vi "GetDisplayName3.vi"(0 "XRef":T15, 1 "State In":T3={"Worker Library Path"=path "", "Block Label"="", "Types"=[], "Selections"=[], "Icon"={"image type"=0, "image depth"=0, "image"=[], "mask"=[], "colors"=[], "Rectangle"={"left"=0, "top"=0, "right"=0, "bottom"=0}}, "Errors"={"Terminals"=[], "Generate"={"status"=FALSE, "code"=0, "source"=""}}, "Calculated Sizes"={"Block Width"=0, "Block Height"=0, "Half Width"=0, "Icon Top"=0, "Icon Bottom"=0, "Label Width"=0, "Half Label"=0, "Label Top"=0, "Text Width"=0, "Half Text"=0, "Text Height"=0, "Label Height"=0, "Expanded Width"=0, "Label Bottom"=0, "Expanded Top"=0, "Expanded Bottom"=0, "Expanded Height"=0, "Min Height"=0, "Max Height"=0}, "Special Terminal Indices"={"Action"=-1, "Init"=-1, "Tag"=-1, "State in"=-1, "State out"=-1, "Error"=-1}, "Terminals"=[]}) -> (14 "Type Name":T2, 15 "Instance Name":T2, 16 "Fatal Error Out":T1)   [LabVIEW 2022 SP3, in "Flex Block.xnode"]
uses:
  Flex Block.xnode
  <vilib>/XNodeSupport/XNodeXNodeRef.ctl
  State.ctl
  FlexBlocks Support/Type Descriptor.ctl
  FlexBlocks Support/Terminal Direction.ctl
  FlexBlocks Support/Value Mode.ctl
  FlexBlocks Support/Special Terminal.ctl
  <vilib>/picture/picture.llb/imagedata.ctl
  FlexBlocks Support/XNode Errors.ctl
  FlexBlocks Support/Calculated Sizes.ctl
  FlexBlocks Support/Special Terminal Indices.ctl
  FlexBlocks Support/Terminal Status.ctl
  FlexBlocks Support/Terminal State.ctl
  FlexBlocks Support/Terminal Draw Style.ctl
  <vilib>/XNodeSupport/XNodeString.ctl
  <vilib>/XNodeSupport/XNodeErrorCluster.ctl
  <vilib>/XNodeSupport/NI_XNodeSupport.lvlib
  FlexBlocks Support/FlexBlocks Support.lvlib
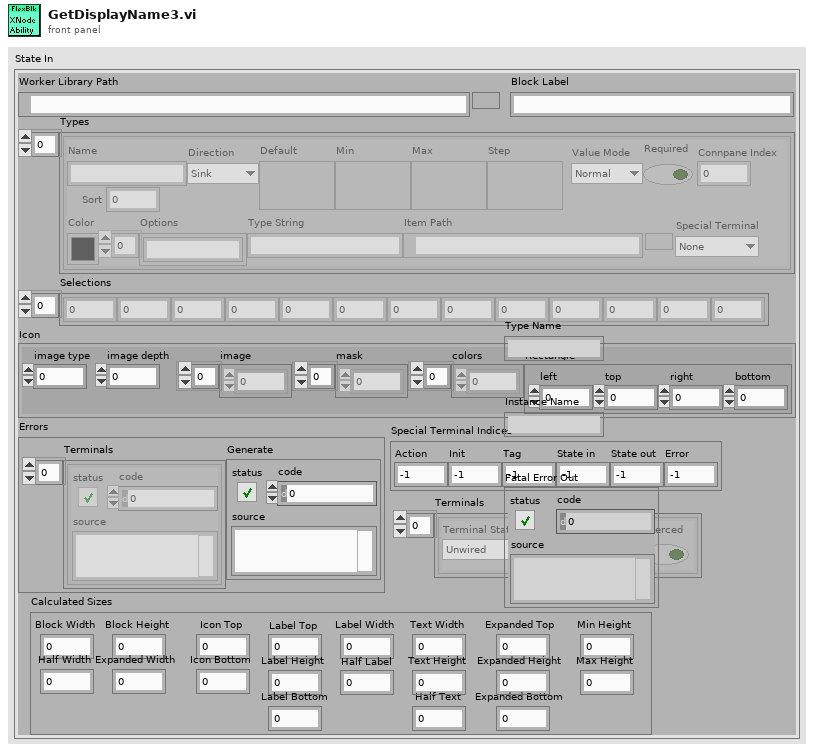
[diagram p1: front panel]
types:
  T1 = typedef "NI_XNodeSupport.lvlib/XNodeErrorCluster.ctl" = errorcluster
  T2 = typedef "NI_XNodeSupport.lvlib/XNodeString.ctl" = string
  T3 = typedef "Flex Block.xnode/State.ctl" = cluster{"Worker Library Path":path, "Block Label":string, "Types":T4[], "Selections":i32[], "Icon":T8, "Errors":T9, "Calculated Sizes":T10, "Special Terminal Indices":T11, "Terminals":T12[]}
  T4 = typedef "FlexBlocks Support.lvlib/Type Descriptor.ctl" = cluster{"Name":string, "Direction":T5, "Default":variant, "Min":variant, "Max":variant, "Step":variant, "Value Mode":T6, "Color":u32, "Options":string[], "Type String":string, "Item Path":path, "Required":bool, "Connpane Index":i32, "Special Terminal":T7, "Sort":i32}
  T5 = typedef "FlexBlocks Support.lvlib/Terminal Direction.ctl" = enum16{"Sink", "Source"}
  T6 = typedef "FlexBlocks Support.lvlib/Value Mode.ctl" = enum16{"Normal", "Range", "Select"}
  T7 = typedef "FlexBlocks Support.lvlib/Special Terminal.ctl" = enum16{"None", "Action", "Init", "Tag", "State in", "State out", "Error"}
  T8 = typedef "imagedata.ctl" = cluster{"image type":i32, "image depth":i32, "image":u8[], "mask":u8[], "colors":u32[], "Rectangle":cluster{"left":i16, "top":i16, "right":i16, "bottom":i16}}
  T9 = typedef "FlexBlocks Support.lvlib/XNode Errors.ctl" = cluster{"Terminals":errorcluster[], "Generate":errorcluster}
  T10 = typedef "FlexBlocks Support.lvlib/Calculated Sizes.ctl" = cluster{"Block Width":i32, "Block Height":i32, "Half Width":i32, "Icon Top":i32, "Icon Bottom":i32, "Label Width":i32, "Half Label":i32, "Label Top":i32, "Text Width":i32, "Half Text":i32, "Text Height":i32, "Label Height":i32, "Expanded Width":i32, "Label Bottom":i32, "Expanded Top":i32, "Expanded Bottom":i32, "Expanded Height":i32, "Min Height":i32, "Max Height":i32}
  T11 = typedef "FlexBlocks Support.lvlib/Special Terminal Indices.ctl" = cluster{"Action":i32, "Init":i32, "Tag":i32, "State in":i32, "State out":i32, "Error":i32}
  T12 = typedef "FlexBlocks Support.lvlib/Terminal Status.ctl" = cluster{"Terminal State":T13, "Draw Style":T14, "Coerced":bool}
  T13 = typedef "FlexBlocks Support.lvlib/Terminal State.ctl" = enum16{"Unwired", "BadType", "BadRef", "Channel", "Value", "Control Ref"}
  T14 = typedef "FlexBlocks Support.lvlib/Terminal Draw Style.ctl" = enum16{"Tunnel", "BadType", "BadRef", "Channel", "Value", "Control Ref"}
  T15 = typedef "NI_XNodeSupport.lvlib/XNodeXNodeRef.ctl" = refnum<vi>
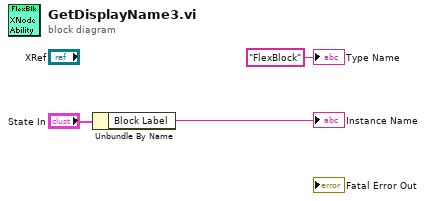
[diagram p0: block diagram]
diagram:
  n1 = Unbundle By Name("State In") -> ("Block Label"=→"Instance Name":string)
  "Type Name" <- T2 "FlexBlock" ("Type Name")
